vi "Station.SetPublishedPages.vi"(8 "error in (no error)":errorcluster, 9 "Pages":string[](array[string]), 10 "Station.ID":string, 11 "state variables in":T1={"Main.DUTs"=[], "Pages.Name"=[], "Pages.Ref"=[], "TS.UI"={"References"={"Event Callback"=refnum, "Quit Application Event"=refnum, "Events"=refnum, "Top level VI"=refnum, "TestStand Engine"=refnum, "Start Application Event"=refnum, "Stop Application Event"=refnum}, "Managers"={"Application Manager"=refnum, "SequenceFileView Manager"=refnum, "ExecutionView Manager"=refnum}, "Controls"={"Execution View"=refnum, "Run Button"=refnum, "Open Button"=refnum}}, "TS.Running"=FALSE, "TS.Abort"=FALSE, "NIVS.GatewayIPAddress"="", "NIVS.WorkspaceManager"=refnum, "NIVS.Open"=FALSE, "NIVS.Deployed"=FALSE, "NIVS.SystemStateRefs"={"CustDatRef"=refnum, "EvtRef"=refnum, "Target State User Event"=refnum}, "NIVS.Events"={"SystemChangeEvent"=refnum, "WorkspaceEvent"=refnum, "WaveformEvent"=refnum}, "UI.Tree"=refnum, "UI.Path"=refnum, "UI.Stop"=refnum, "UI.Tab"=refnum, "VI.Ref"=refnum, "Analysis.Parameters"={"Global.ResultsPath"=path "C:/testdata/Logs", "Global.TempPath"=path "C:/testdata/Temp", "Global.RemotePath"=path "d:/testdata/Logs", "TDMS.AnalysisVIs"=[path "C:/addons/TestStand Examples for HIL/Continuous Monitoring Tester/TestStand Sequences/LabVIEW Steps/Builds/TestStand Analysis Steps.lvlibp/Post Process Analysis Steps/Analysis.LevelTransition.vi"], "TDMS.ReportPassed"=TRUE, "TDMS.GroupChannels"=TRUE}, "DUTExecution.Tabs"=[], "Overview.Columns"=[], "SharedExecution.Tabs"=[], "SharedExecution.Use"=TRUE}) -> (0 "error out":errorcluster)   [LabVIEW 2015, in "Main.GUI.lvlib"]
uses:
  Main.GUI.lvlib
  Types/Multihead.StateVariables.ctl
  Types/TestStandGUI.Refs.ctl
  <vilib>/NI Veristand/Execution/Workspace/WorkspaceAPI.ctl
  NationalInstruments.VeriStand.ClientAPI
  <vilib>/NI Veristand/Execution/Workspace/SystemStateEventRef.ctl
  <vilib>/NI Veristand/Execution/Workspace/Target State Info.ctl
  <vilib>/NI Veristand/Execution/Workspace/Target State.ctl
  Execution GUI/Types/Execute.UserEventRefs.ctl
  <vilib>/NI Veristand/Execution/Workspace/SystemStateRegEventRef.ctl
  <vilib>/NI Veristand/Execution/WaveformStreaming/Waveform Data Watcher Event Data (DBL).ctl
  <vilib>/NI Veristand/Execution/WaveformStreaming/WaveformStreamSpecification.ctl
  Analysis GUI/Types/Analysis.GUI.Parameters.ctl
  <vilib>/NI Veristand/Execution/Workspace/NI_VS Workspace ExecutionAPI.lvlib
  <vilib>/NI Veristand/Execution/WaveformStreaming/NI_VS Waveform Streaming Interface.lvlib
  Execution GUI/Station.Execution.lvlib
  Analysis GUI/Analysis.lvlib
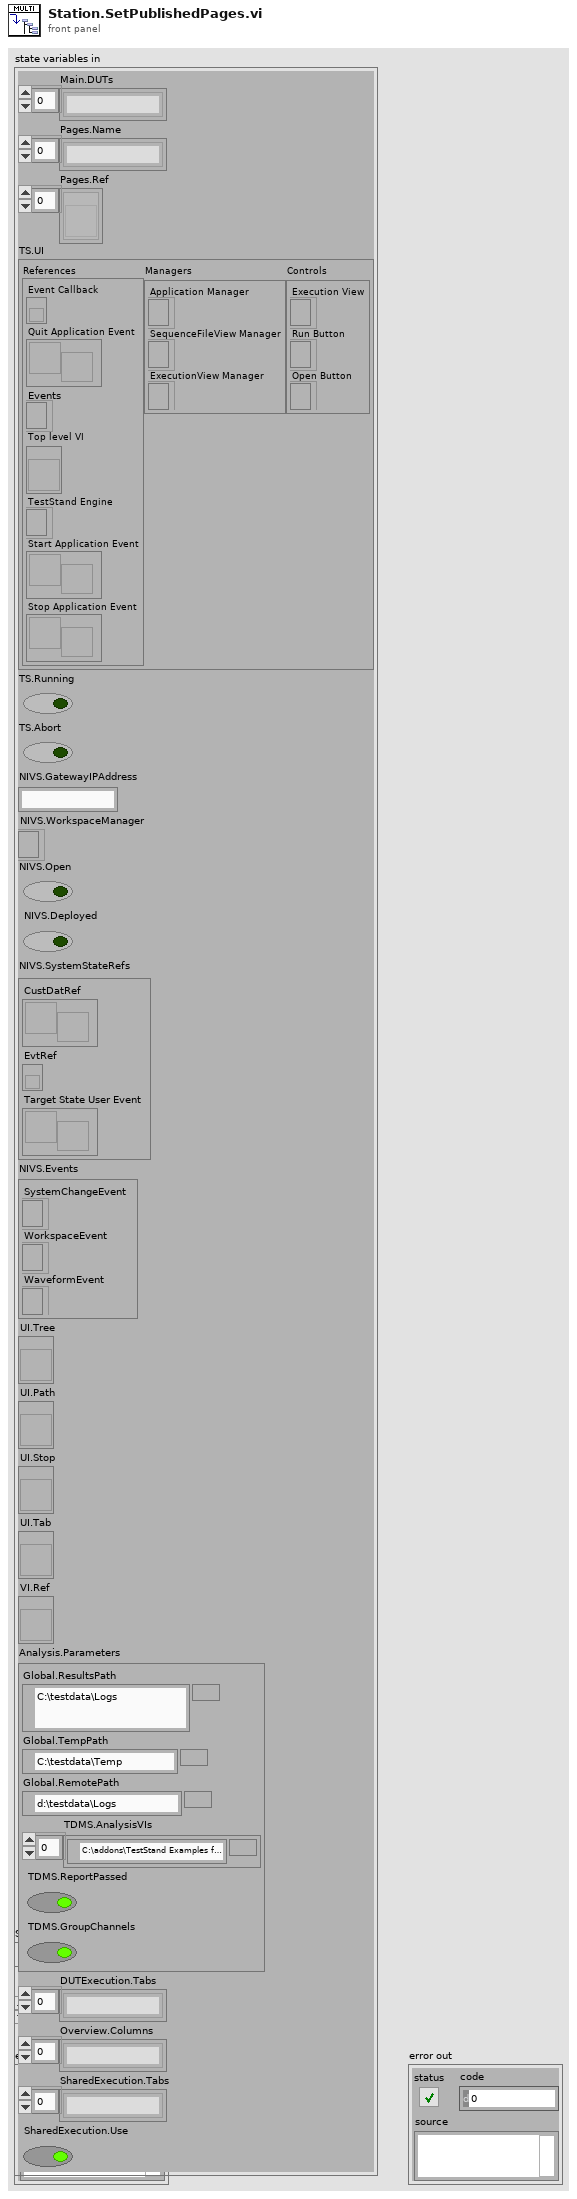
[diagram p1: front panel]
types:
  T1 = typedef "Main.GUI.lvlib/Multihead.StateVariables.ctl" = cluster{"Main.DUTs":string[], "Pages.Name":string[], "Pages.Ref":refnum<vi>[], "TS.UI":T2, "TS.Running":bool, "TS.Abort":bool, "NIVS.GatewayIPAddress":string, "NIVS.WorkspaceManager":T3, "NIVS.Open":bool, "NIVS.Deployed":bool, "NIVS.SystemStateRefs":T4, "NIVS.Events":T5, "UI.Tree":refnum<vi>, "UI.Path":refnum<vi>, "UI.Stop":refnum<vi>, "UI.Tab":refnum<vi>, "VI.Ref":refnum<vi>, "Analysis.Parameters":T7, "DUTExecution.Tabs":string[], "Overview.Columns":string[], "SharedExecution.Tabs":string[], "SharedExecution.Use":bool}
  T2 = typedef "Main.GUI.lvlib/TestStandGUI.Refs.ctl" = cluster{"References":cluster{"Event Callback":refnum<k27>, "Quit Application Event":refnum<user-event>, "Events":refnum<event-registration>, "Top level VI":refnum<vi>, "TestStand Engine":refnum<k7>, "Start Application Event":refnum<user-event>, "Stop Application Event":refnum<user-event>}, "Managers":cluster{"Application Manager":refnum<k7>, "SequenceFileView Manager":refnum<k7>, "ExecutionView Manager":refnum<k7>}, "Controls":cluster{"Execution View":refnum<k7>, "Run Button":refnum<k7>, "Open Button":refnum<k7>}}
  T3 = typedef "NI_VS Workspace ExecutionAPI.lvlib/WorkspaceAPI.ctl" = refnum<k24>
  T4 = typedef "NI_VS Workspace ExecutionAPI.lvlib/SystemStateEventRef.ctl" = cluster{"CustDatRef":refnum<user-event>, "EvtRef":refnum<k27>, "Target State User Event":refnum<user-event>}
  T5 = typedef "Station.Execution.lvlib/Execute.UserEventRefs.ctl" = cluster{"SystemChangeEvent":T6, "WorkspaceEvent":refnum<event-registration>, "WaveformEvent":refnum<event-registration>}
  T6 = typedef "NI_VS Workspace ExecutionAPI.lvlib/SystemStateRegEventRef.ctl" = refnum<event-registration>
  T7 = typedef "Analysis.lvlib/Analysis.GUI.Parameters.ctl" = cluster{"Global.ResultsPath":path, "Global.TempPath":path, "Global.RemotePath":path, "TDMS.AnalysisVIs":path[], "TDMS.ReportPassed":bool, "TDMS.GroupChannels":bool}
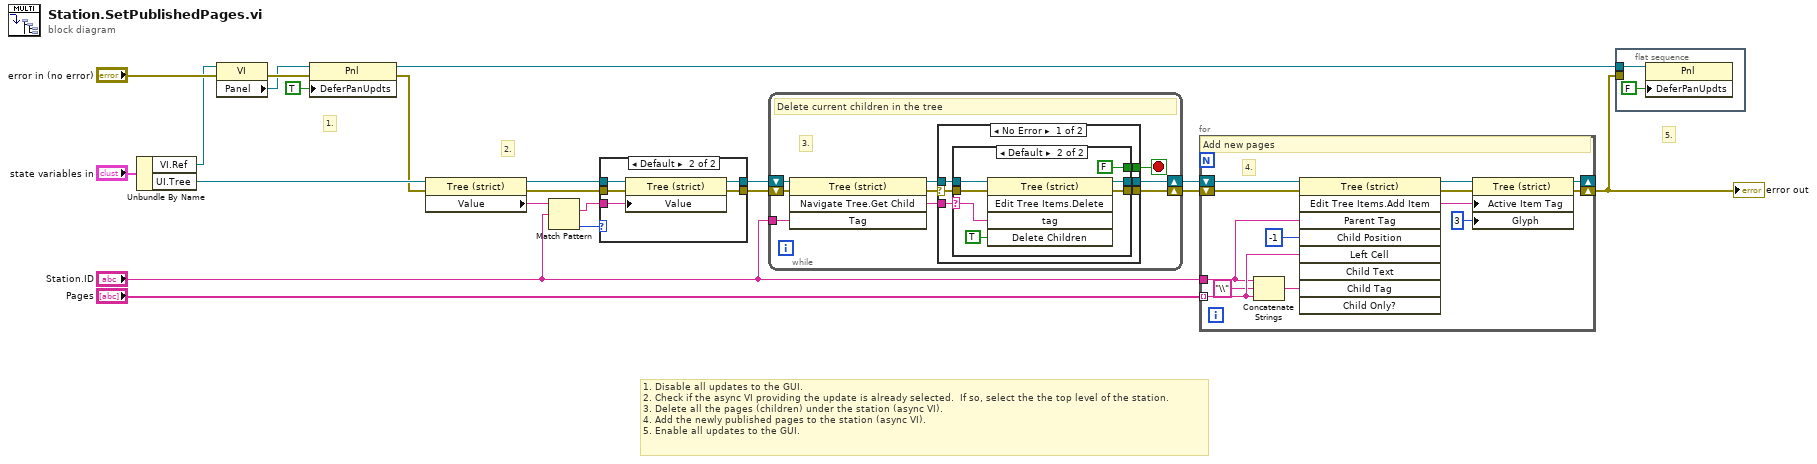
[diagram p0: block diagram]
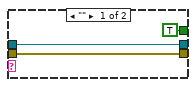
[diagram p3: hidden frame]
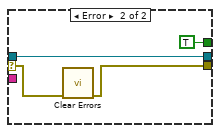
[diagram p4: hidden frame]
diagram:
  # "1. Disable all updates to the GUI.\n2. Check if the async VI providing the update is already selected.  If so, select the the top level of the station.\n3. Delete all the pages (children) under the station (async VI).\n4. Add the newly published pages to the station (async VI).\n5. Enable all updates to the GUI."
  # "5."
  # "2."
  # "1."
  n1 = Unbundle By Name("state variables in") -> ("VI.Ref"=w13:refnum<vi>, "UI.Tree"=w17:refnum<vi>)
  n2 = property class="VI"(reference=w13, error in="error in (no error)") -> (error out=w11:errorcluster, "Panel"=w10:refnum<vi>)  [unwired: 1 out]
  n3 = property class="Pnl"(reference=w10, error in=w11, "DeferPanUpdts"=TRUE ("Defer Panel Updates")) -> (reference out=w14:refnum<vi>, error out=w3:errorcluster)
  n4 = property class="Tree (strict)"(reference=w17, error in=w3) -> (reference out=w21:refnum<vi>, error out=w4:errorcluster, "Value"=w18:string)
  n5 = Match Pattern(string=w18, regular expression="Station.ID") -> (match substring=w5:string, offset past match=w19:i32)  [unwired: 1 in, 2 out]
  n6 = case shown="Default" w19 {
    tunnel: w5 -> [_ w28]
    tunnel: w21 -> [w22 w27]
    tunnel: w4 -> [w23 w26]
    tunnel: [w23 w25] -> w2
    tunnel: [w22 w24] -> w1
    frame -1 {
    }
    frame Default {
      n7 = property class="Tree (strict)"(reference=w27, error in=w26, "Value"=w28) -> (reference out=w24:refnum<vi>, error out=w25:errorcluster)
    }
  }
  n8 = while {
    tunnel: "Station.ID" -> [w35]
    shift-right: [w36] -> w7
    shift-left: w2 -> [w37]
    shift-right: [w31] -> w8
    shift-left: w1 -> [w30]
    stop <- w34 stop-if-true
    # "3."
    # "Delete current children in the tree"
    n9 = invoke class="Tree (strict)" method="Navigate Tree.Get Child"(reference=w30, error in=w37, "Tag"=w35) -> (reference out=w33:refnum<vi>, error out=w29:errorcluster, "Navigate Tree:Get Child"=w32:string)  [unwired: 1 in, 1 out]
    n10 = case shown="No Error" w29 {
      selector: w29 -> [w38 w55]
      tunnel: [w43 w54] -> w36
      tunnel: [w42 TRUE] -> w34
      tunnel: w33 -> [w41 w56]
      tunnel: w32 -> [w40 _]
      tunnel: [w39 w56] -> w31
      frame No Error {
        n11 = case shown="Default" w40 {
          selector: w40 -> [_ w48]
          tunnel: [w46 w53] -> w43
          tunnel: [TRUE FALSE] -> w42
          tunnel: w41 -> [w44 w51]
          tunnel: w38 -> [w46 w50]
          tunnel: [w44 w47] -> w39
          frame "" {
          }
          frame Default {
            n12 = invoke class="Tree (strict)" method="Edit Tree Items.Delete"(reference=w51, error in=w50, "tag"=w48, "Delete Children"=TRUE ("Delete Children?")) -> (reference out=w47:refnum<vi>, error out=w53:errorcluster)  [unwired: 1 in, 3 out]
          }
        }
      }
      frame Error {
        n13 = call <vilib>:"Clear Errors.vi"("error in (no error)"=w55) -> ("error out"=w54:errorcluster)  [unwired: 5 in, 1 out]
      }
    }
  }
  n14 = for {
    tunnel: "Pages" -> [w69] mode=indexing
    shift-right: [w59] -> w16
    shift-left: w7 -> [w70]
    tunnel: "Station.ID" -> [w65]
    shift-right: [w58] -> _
    shift-left: w8 -> [w66]
    # "4."
    # "Add new pages"
    n15 = Concatenate Strings(w65, "\\" ("string"), w69) -> (w68:string)
    n16 = invoke class="Tree (strict)" method="Edit Tree Items.Add Item"(reference=w66, error in=w70, "Parent Tag"=w65, "Child Position"=-1, "Left Cell"=w69, "Child Tag"=w68) -> (reference out=w61:refnum<vi>, error out=w60:errorcluster, "Edit Tree Items:Add Item"=w62:string)  [unwired: 3 in, 6 out]
    n17 = property class="Tree (strict)"(reference=w61, error in=w60, "Active Item Tag"=w62, "Glyph"=3 ("Active Item:Symbol Index")) -> (reference out=w58:refnum<vi>, error out=w59:errorcluster)
  }
  "error out" <- w16
  n18 = flat-sequence {
    tunnel: w14 -> [w72]
    tunnel: w16 -> [_]
    frame #0 {
      n19 = property class="Pnl"(reference=w72, "DeferPanUpdts"=FALSE ("Defer Panel Updates")) -> ()  [unwired: 1 in, 2 out]
    }
  }
